vi "Generate Signal.vi"(0 "noise amplitude":u16, 5 "frequency (periods/tick)":fxp<+,32,0>=0.0002500000409781933, 7 "DC offset":fxp<+/-,16,5>) -> (4 "signal":fxp<+/-,16,5>)   [LabVIEW 2020]
doc: "This VI generates a +-8.19V sine tone with adjustable DC offset and uniform noise."
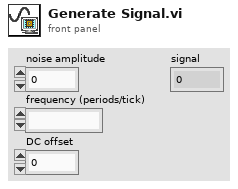
[diagram p1: front panel]
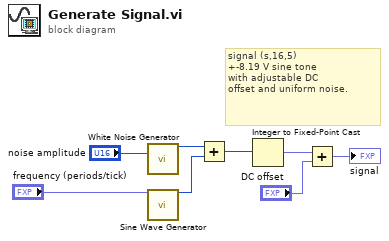
[diagram p0: block diagram]
diagram:
  # "signal (s,16,5)\n+-8.19 V sine tone\nwith adjustable DC\noffset and uniform noise."
  n1 = call "White Noise Generator"("amplitude"="noise amplitude") -> ("white noise out"=w8:i16)  [unwired: 14 in]
  n2 = call "Sine Wave Generator"("frequency (periods/tick)"="frequency (periods/tick)") -> ("sine out"=w7:i16)  [unwired: 14 in]
  n3 = Add(x=w8, y=w7) -> (x+y=w2:i16)
  n4 = Integer to Fixed-Point Cast(integer=w2) -> (fixed-point=w1:fxp<+/-,16,5>)  [unwired: 1 in]
  n5 = Add(x=w1, y="DC offset") -> (x+y=→"signal":fxp<+/-,16,5>)
